vi "Do Action.vi"(4 "error in (no error)":errorcluster, 6 "Array in":refnum<class>[](array[class]), 7 "Act_Delete All in":refnum<class "Act_Delete All.lvclass">) -> (0 "error out":errorcluster, 2 "Array out":refnum<class>[](array[class]), 3 "Act_Delete All out":refnum<class "Act_Delete All.lvclass">)   [LabVIEW 2014, in "Act_Delete All.lvclass"]
uses:
  Act_Delete All.lvclass
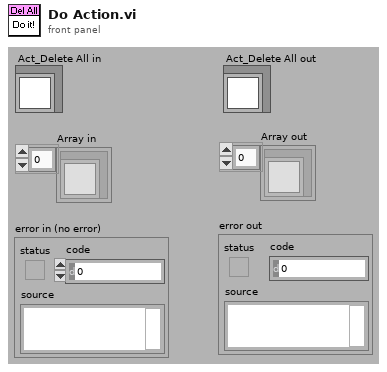
[diagram p1: front panel]
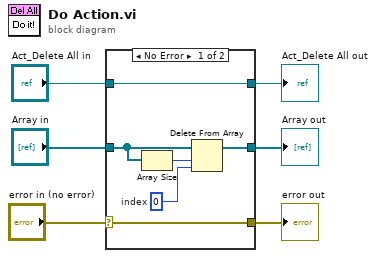
[diagram p0: block diagram]
diagram:
  n1 = case shown="No Error" "error in (no error)" {
    selector: "error in (no error)" -> [w12 w13]
    tunnel: [w12 w13] -> w5
    tunnel: [w11 w15] -> w4
    tunnel: "Act_Delete All in" -> [w11 w15]
    tunnel: [w10 w14] -> w2
    tunnel: "Array in" -> [w7 w14]
    frame No Error {
      w9 = 0  # index
      n2 = Array Size(array=w7) -> (size(s)=w8:i32)
      n3 = Delete From Array(array=w7, length=w8, index=w9) -> (array with subset deleted=w10:refnum<class>[])  [unwired: 1 out]
    }
    frame Error {
    }
  }
  "error out" <- w5
  "Array out" <- w2
  "Act_Delete All out" <- w4
